vi "Button Text Read.vi"(4 "error in (no error)":errorcluster, 6 "Container State":T2, 7 "Display State In":T1) -> (0 "error out":errorcluster, 2 "Value":string, 3 "Display State Out":T1)   [LabVIEW 2009, in "Next Button (System).xctl"]
uses:
  <vilib>/Navigation Controls/Next Button System/Next Button (System).xctl
  <vilib>/_xctls/Container State.ctl
  <vilib>/Navigation Controls/Next Button System/Next Button State.ctl
  <vilib>/_xctls/XControlSupport.lvlib
panel:
  # "Replace the Value Indicator below with an Indicator of desired type.\nDo not remove this Indicator or the others from the connector pane. \nDo not change the connector pane pattern.\nThe Value Indicator should always be the second terminal from top on the output side in the connector pane."
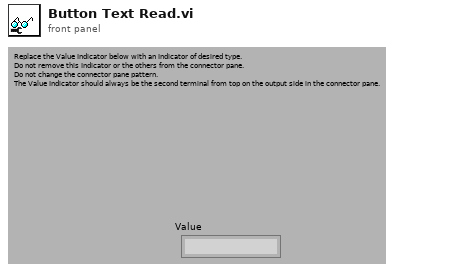
[diagram p1: front panel]
types:
  T1 = typedef "Next Button (System).xctl/Next Button State.ctl" = cluster{"Button Text":string}
  T2 = typedef "XControlSupport.lvlib/Container State.ctl" = cluster{"Indicator?":bool, "Run Mode?":bool, " Refnum":refnum<vi>}
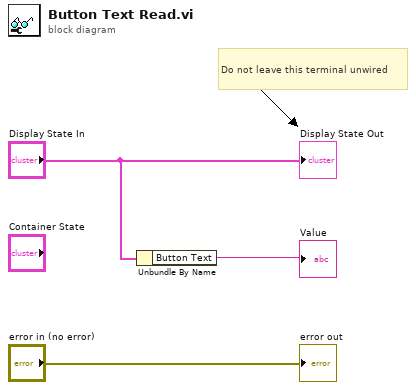
[diagram p0: block diagram]
diagram:
  # "Do not leave this terminal unwired"
  n1 = Unbundle By Name("Display State In") -> ("Button Text"=→"Value":string)
  "error out" <- "error in (no error)"
  "Display State Out" <- "Display State In"
